vi "create_table.vi"(8 "error in (no error)":errorcluster, 10 "Table Name":string, 11 "Doc in":refnum<class "Doc.lvclass">) -> (0 "error out":errorcluster, 3 "Doc out":refnum<class "Doc.lvclass">)   [LabVIEW 2020]
uses:
  Doc.lvclass/Doc.ctl
  Doc.lvclass
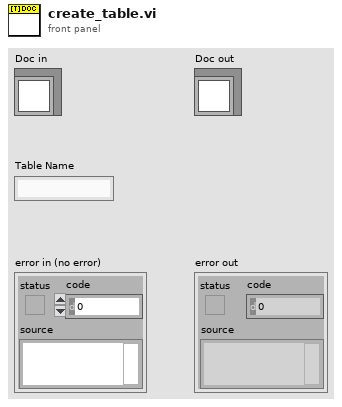
[diagram p1: front panel]
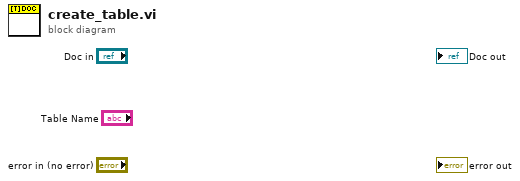
[diagram p0: block diagram]
diagram:
